vi "PH_Names.Instance Name Manipulator.vi"(3 "error in (no error)":errorcluster, 5 "name in":string) -> (0 "error out":errorcluster, 1 "systemID":string, 2 "name out":string)   [LabVIEW 2014, in "PH_Common.lvlib"]
doc: "This VI checks wether <name in> contains the current system ID; if so, nothing is done. Else, the system ID is set before the name on order to get a manipulated <name out> as <system ID>\\<name in>."
uses:
  PH_Common.lvlib
  CSCore/CSSystem/CSSystemLib/CSSystemLib.lvlib
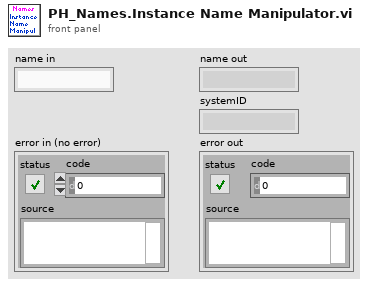
[diagram p1: front panel]
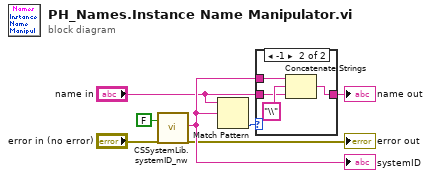
[diagram p0: block diagram]
diagram:
  n1 = call "CSSystemLib.systemID_nw.vi"("set ID"=FALSE, "error in (no error)"="error in (no error)") -> ("systemID out"=w6:string, "error out"=→"error out":errorcluster)  [unwired: 16 in]
  "systemID" <- w6
  n2 = Match Pattern(string="name in", regular expression=w6) -> (offset past match=w7:i32)  [unwired: 1 in, 3 out]
  n3 = case shown="-1" w7 {
    tunnel: [w8 w11] -> w4
    tunnel: "name in" -> [w8 w10]
    tunnel: w6 -> [_ w9]
    frame Default {
    }
    frame -1 {
      n4 = Concatenate Strings(w9, "\\" ("string"), w10) -> (w11:string)
    }
  }
  "name out" <- w4
